vi "Write a frame to the acquisition file.vi"(1 "Pixel depth":u32(ring) items=["8 bits", "16 bits", "Float", "Complex", "RGB", "HSL"], 4 "Frames per acquisition file":u32, 7 "Offset table in":T2, 8 "error in":errorcluster, 9 "Image In":T5, 10 "Sequence files handle":T1, 11 "Last frame number written in":u32) -> (0 "error out":errorcluster, 2 "Last frame number written out":u32, 3 "Stop":bool, 5 "Offset table out":T2)   [LabVIEW 2016]
uses:
  <vilib>/vision/Image Controls.llb/IMAQ Image.ctl
  Seq file v 1/Offset table.ctl
  Seq file v 1/Offset.ctl
  Seq file v 1/file number.ctl
  Sequence files handle.ctt
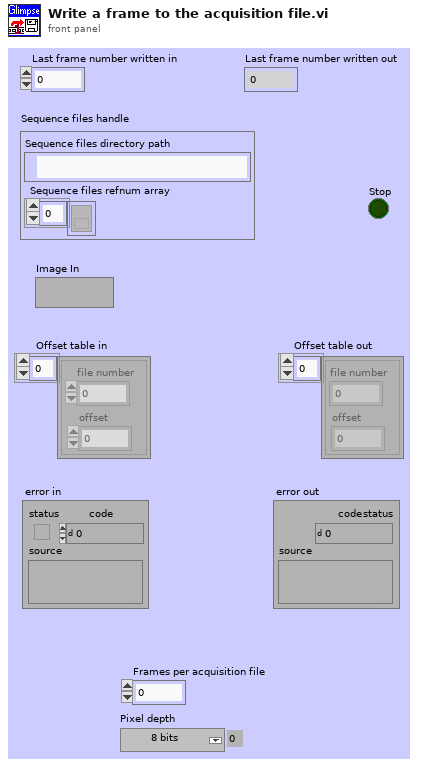
[diagram p1: front panel]
types:
  T1 = typedef "Sequence files handle.ctt" = cluster{"Sequence files directory path":path, "Sequence files refnum array":refnum<file>[]}
  T2 = typedef "Offset table.ctl" = cluster{"offset":T3, "file number":T4}[]
  T3 = typedef "Offset.ctl" = i32
  T4 = typedef "file number.ctl" = u8
  T5 = typedef "IMAQ Image.ctl" = refnum<image>
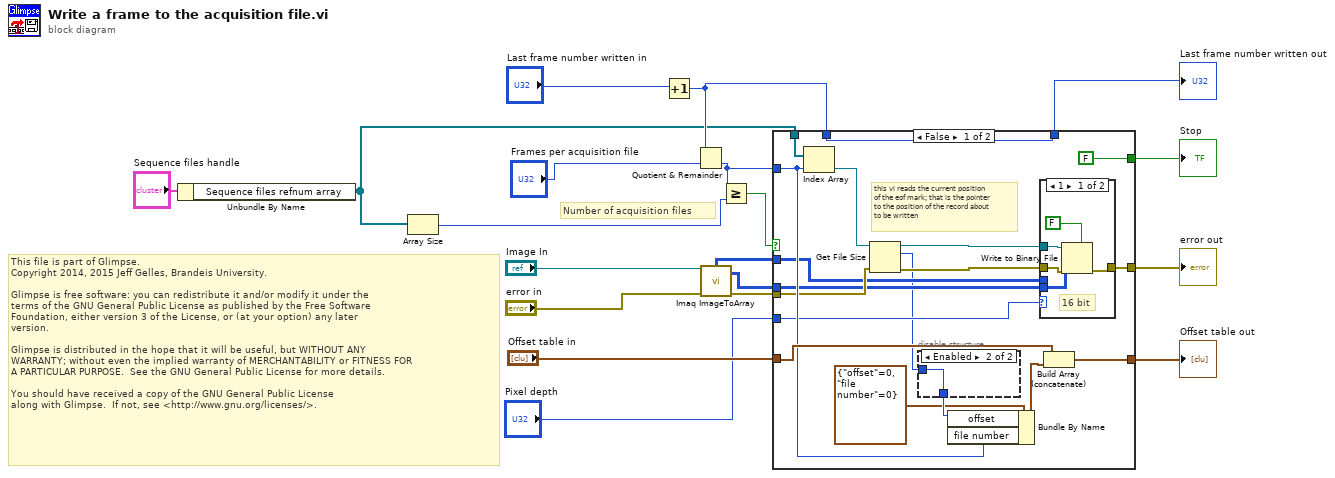
[diagram p0: block diagram]
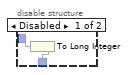
[diagram p2: hidden frame]
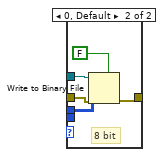
[diagram p3: hidden frame]
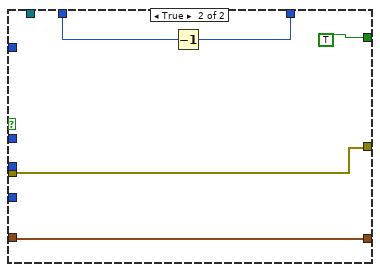
[diagram p4: hidden frame]
diagram:
  # "This file is part of Glimpse. \nCopyright 2014, 2015 Jeff Gelles, Brandeis University.    \n\nGlimpse is free software: you can redistribute it and/or modify it under the \nterms of the GNU General Public License as published by the Free Software \nFoundation, either version 3 of the License, or (at your option) any later \nversion.\n\nGlimpse is distributed in the hope that it will be useful, but WITHOUT ANY \nWARRANTY; without even the implied warranty of MERCHANTABILITY or FITNESS FOR \nA PARTICULAR PURPOSE.  See the GNU General Public License for more details.\n\nYou should have received a copy of the GNU General Public License\nalong with Glimpse.  If not, see <http://www.gnu.org/licenses/>."
  # "Number of acquisition files"
  n1 = Unbundle By Name("Sequence files handle") -> ("Sequence files refnum array"=w1:refnum<file>[])
  n2 = Array Size(array=w1) -> (size(s)=w3:i32)
  n3 = Increment(x="Last frame number written in") -> (x+1=w15:u32)
  n4 = Quotient & Remainder(x=w15, y="Frames per acquisition file") -> (floor(x/y)=w13:u32)  [unwired: 1 out]
  n5 = call "Imaq ImageToArray"("error in (no error)"="error in", "Image"="Image In") -> ("error out"=w10:errorcluster, "Image Pixels (U8)"=w11:u8[][], "Image Pixels (I16)"=w6:i16[][])  [unwired: 1 in, 3 out]
  n6 = Greater Or Equal?(x=w13, y=w3) -> (x >= y?=w16:bool)
  n7 = case shown="False" w16 {
    tunnel: w15 -> [w35 w55]
    tunnel: [w35 w54] -> w14
    tunnel: w1 -> [w37 _]
    tunnel: w13 -> [w30 _]
    tunnel: [FALSE TRUE] -> w12
    tunnel: w11 -> [w24 _]
    tunnel: w10 -> [w27 w52]
    tunnel: [w34 w52] -> w9
    tunnel: "Offset table in" -> [w33 w51]
    tunnel: [w31 w51] -> w7
    tunnel: w6 -> [w23 _]
    tunnel: "Pixel depth" -> [w22 _]
    frame False {
      # "this vi reads the current position\nof the eof mark; that is the pointer\nto the position of the record about\nto be written"
      n8 = Index Array(array=w37, index=w30) -> (element=w29:refnum<file>)
      n9 = Get File Size(file=w29, error in=w27) -> (refnum out=w28:refnum<file>, size (in bytes)=w21:i64, 0:w26:errorcluster)
      n10 = disable-structure shown="Enabled" {
        disable-tunnel: [w39 w40] -> w25
        disable-tunnel: w21 -> [w38 w40]
        frame Disabled {
          n11 = To Long Integer(number=w38) -> (32bit integer=w39:i32)
        }
        frame Enabled {
        }
      }
      n12 = Bundle By Name(cluster=cluster{"offset":T3, "file number":T4} {"offset"=0, "file number"=0} ("Cluster"), "offset"=w25, "file number"=w30) -> (w32:cluster{"offset":T3, "file number":T4})
      n13 = case shown="1" w22 {
        tunnel: [w45 w50] -> w34
        tunnel: w28 -> [w44 w49]
        tunnel: w26 -> [w43 w48]
        tunnel: w24 -> [_ w47]
        tunnel: w23 -> [w42 _]
        frame 1 {
          # "16 bit"
          n14 = Write to Binary File(file (use dialog)=w44, data=w42, error in=w43, 5:FALSE ("prepend array or string size? (T)")) -> (error out=w45:errorcluster)  [unwired: 4 out]
        }
        frame 0, Default {
          # "8 bit"
          n15 = Write to Binary File(file (use dialog)=w49, data=w47, error in=w48, 5:FALSE ("prepend array or string size? (T)")) -> (error out=w50:errorcluster)  [unwired: 4 out]
        }
      }
      n16 = Build Array (concatenate)(w33, w32) -> (w31:T2)
    }
    frame True {
      n17 = Decrement(x=w55) -> (x-1=w54:u32)
    }
  }
  "Last frame number written out" <- w14
  "error out" <- w9
  "Stop" <- w12
  "Offset table out" <- w7
